vi "Set Clusters Visibility.vi"(4 "Normal Operation Control Cluster":refnum<vi>, 5 "Connection Status":T2, 6 "Connection Configuration Cluster":refnum<vi>, 8 "Error In":errorcluster, 9 "Control Type":T1, 10 "Normal Operation Indicator Cluster":refnum<vi>) -> (0 "Error Out":errorcluster, 1 "User Help":string, 3 "Control Type Out":T1)   [LabVIEW 2014]
doc: "Sets clusters visibility according to chosen mode for normal operation"
uses:
  Controls/Connection Status.ctl
  Controls/Controllers.ctl
  Controls/Controllers Clusters/Normal Operation Indicator Cluster.ctl
  Controls/User Help.ctl
  Controls/Controllers Clusters/Order in Normal Operation Control Cluster.ctl
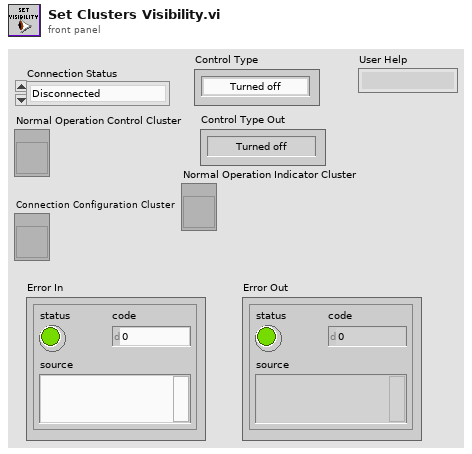
[diagram p1: front panel]
types:
  T1 = typedef "Controllers.ctl" = enum16{"Turned off", "Keyboard", "Mouse", "Pad", "Autonomous"}
  T2 = typedef "Connection Status.ctl" = enum16{"Disconnected", "Connected"}
  T3 = typedef "User Help.ctl" = enum16{"The Reaper Controller says hello!\nFirst you should establish connection with The Reaper.", "Connection established! Choose control mode.", "Something went wrong. Try another COM port.", "Disconnected. Do you want to connect again?", "Controls turned off", "Keyboard Mode", "Mouse Mode", "Pad Mode", "Autonomous Mode", "Unknown Operation occured", "Please connect before choosing control type!", "Settings available only if disconnected.", "Settings updated."}
  T4 = typedef "Order in Normal Operation Control Cluster.ctl" = enum16{"Disconnect Button", "Select Controller", "General Control Cluster ", "Game Pad Indicator Cluster", "Game Pad Control Cluster", "Mouse Control Cluster"}
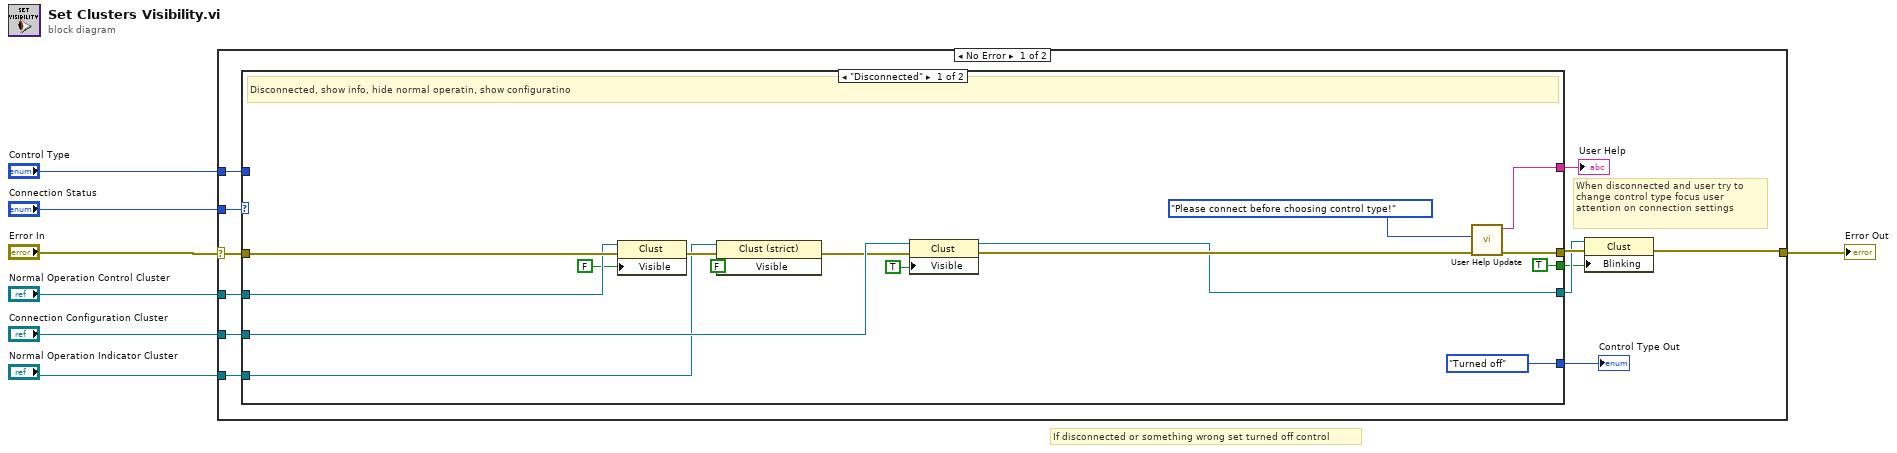
[diagram p0: block diagram]
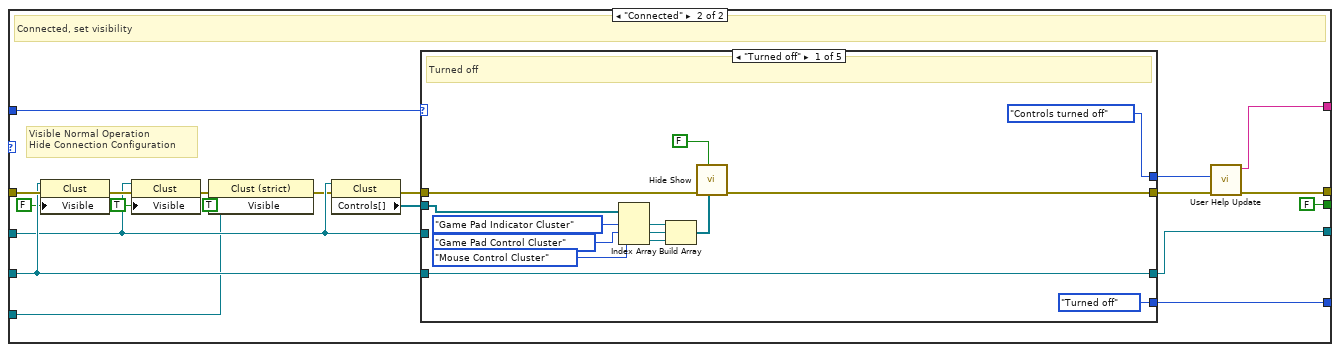
[diagram p2: hidden frame]
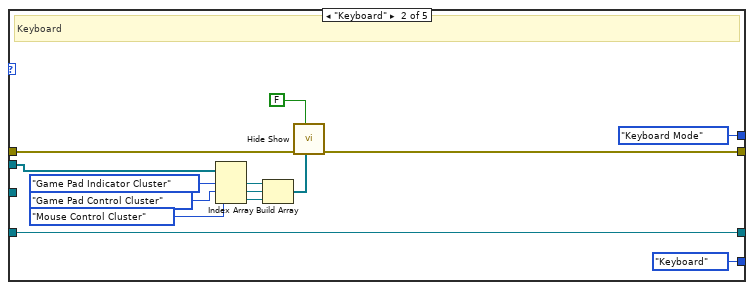
[diagram p3: hidden frame]
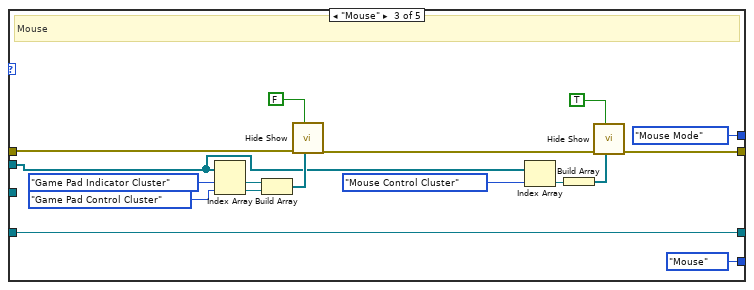
[diagram p4: hidden frame]
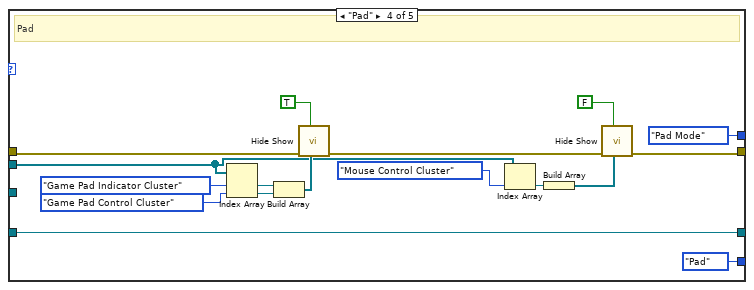
[diagram p5: hidden frame]
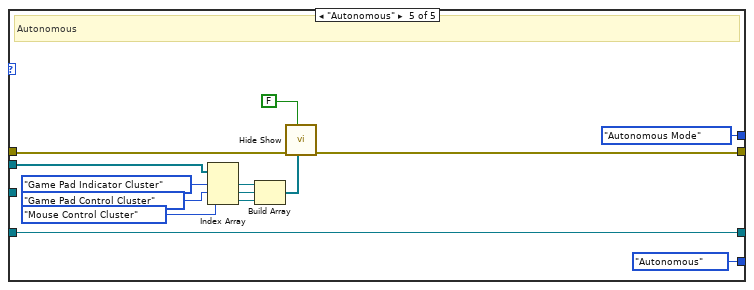
[diagram p6: hidden frame]
diagram:
  # "If disconnected or something wrong set turned off control"
  n1 = case shown="No Error" "Error In" {
    selector: "Error In" -> [w18 w132]
    tunnel: [w12 w132] -> w6
    tunnel: "Control Type" -> [w17 _]
    tunnel: "Connection Status" -> [w19 _]
    tunnel: "Normal Operation Control Cluster" -> [w16 _]
    tunnel: "Connection Configuration Cluster" -> [w15 _]
    tunnel: "Normal Operation Indicator Cluster" -> [w8 _]
    frame No Error {
      # "When disconnected and user try to change control type focus user attention on connection settings"
      n2 = case shown="\"Disconnected\"" w19 {
        tunnel: [w29 w53] -> w13
        tunnel: w18 -> [w35 w48]
        tunnel: w17 -> [_ w55]
        tunnel: w16 -> [w33 w42]
        tunnel: w15 -> [w34 w46]
        tunnel: [w30 w52] -> w14
        tunnel: [w26 w49] -> w11
        tunnel: [TRUE FALSE] -> w10
        tunnel: [Controllers."Turned off" ("Control Type") w43] -> w9
        tunnel: w8 -> [w20 w39]
        frame "Disconnected" {
          # "Disconnected, show info, hide normal operatin, show configuratino"
          n3 = property class="Clust"(reference=w33, error in=w35, "Visible"=FALSE) -> (error out=w23:errorcluster)  [unwired: 1 out]
          n4 = property class="Clust (strict)"(reference=w20, error in=w23, "Visible"=FALSE) -> (error out=w22:errorcluster)  [unwired: 1 out]
          n5 = property class="Clust"(reference=w34, error in=w22, "Visible"=TRUE) -> (reference out=w26:refnum<vi>, error out=w27:errorcluster)
          n6 = call "User Help Update.vi"("Error In"=w27, "Enum"=User_Help."Please connect before choosing control type!") -> ("Error Out"=w29:errorcluster, "User Help Out"=w30:string)  [unwired: 8 in]
        }
        frame "Connected" {
          # "Visible Normal Operation\nHide Connection Configuration"
          # "Connected, set visibility"
          n7 = property class="Clust"(reference=w46, error in=w48, "Visible"=FALSE) -> (error out=w47:errorcluster)  [unwired: 1 out]
          n8 = property class="Clust"(reference=w42, error in=w47, "Visible"=TRUE) -> (error out=w37:errorcluster)  [unwired: 1 out]
          n9 = property class="Clust (strict)"(reference=w39, error in=w37, "Visible"=TRUE) -> (error out=w36:errorcluster)  [unwired: 1 out]
          n10 = property class="Clust"(reference=w42, error in=w36) -> (error out=w41:errorcluster, "Controls[]"=w40:refnum<vi>[])  [unwired: 1 out]
          n11 = case shown="\"Turned off\"" w55 {
            tunnel: [w60 w75 w90 w106 w123] -> w54
            tunnel: w41 -> [w66 w76 w93 w110 w124]
            tunnel: w42 -> [_ _ _ _ _]
            tunnel: [User_Help."Controls turned off" ("Enum") User_Help."Keyboard Mode" ("Enum") User_Help."Mouse Mode" ("Enum") User_Help."Pad Mode" ("Enum") User_Help."Autonomous Mode" ("Enum")] -> w51
            tunnel: [w68 w82 w99 w116 w130] -> w49
            tunnel: w46 -> [w68 w82 w99 w116 w130]
            tunnel: [Controllers."Turned off" ("Control Type") Controllers."Keyboard" ("Control Type") Controllers."Mouse" ("Control Type") Controllers."Pad" ("Control Type") Controllers."Autonomous" ("Control Type")] -> w43
            tunnel: w40 -> [w65 w74 w85 w104 w122]
            frame "Turned off" {
              # "Turned off"
              n12 = Index Array(array=w65, index #1=Order_in_Normal_Operation_Control_Cluster."Game Pad Indicator Cluster" ("Order in Normal Operation Control Cluster"), index #2=Order_in_Normal_Operation_Control_Cluster."Game Pad Control Cluster" ("Order in Normal Operation Control Cluster"), index #3=Order_in_Normal_Operation_Control_Cluster."Mouse Control Cluster" ("Order in Normal Operation Control Cluster")) -> (element #1=w63:refnum<vi>, element #2=w58:refnum<vi>, element #3=w57:refnum<vi>)
              n13 = Build Array(w63, w58, w57) -> (w62:refnum<vi>[])
              n14 = call "Hide Show.vi"("Controls[]"=w62, "Visible?"=FALSE, "Error In"=w66) -> ("Error Out"=w60:errorcluster)  [unwired: 8 in]
            }
            frame "Keyboard" {
              # "Keyboard"
              n15 = Index Array(array=w74, index #1=Order_in_Normal_Operation_Control_Cluster."Game Pad Indicator Cluster" ("Order in Normal Operation Control Cluster"), index #2=Order_in_Normal_Operation_Control_Cluster."Game Pad Control Cluster" ("Order in Normal Operation Control Cluster"), index #3=Order_in_Normal_Operation_Control_Cluster."Mouse Control Cluster" ("Order in Normal Operation Control Cluster")) -> (element #1=w79:refnum<vi>, element #2=w72:refnum<vi>, element #3=w70:refnum<vi>)
              n16 = Build Array(w79, w72, w70) -> (w78:refnum<vi>[])
              n17 = call "Hide Show.vi"("Controls[]"=w78, "Visible?"=FALSE, "Error In"=w76) -> ("Error Out"=w75:errorcluster)  [unwired: 8 in]
            }
            frame "Mouse" {
              # "Mouse"
              n18 = Index Array(array=w85, index #1=Order_in_Normal_Operation_Control_Cluster."Game Pad Indicator Cluster" ("Order in Normal Operation Control Cluster"), index #2=Order_in_Normal_Operation_Control_Cluster."Game Pad Control Cluster" ("Order in Normal Operation Control Cluster")) -> (element #1=w96:refnum<vi>, element #2=w91:refnum<vi>)
              n19 = Build Array(w96, w91) -> (w95:refnum<vi>[])
              n20 = call "Hide Show.vi"("Controls[]"=w95, "Visible?"=FALSE, "Error In"=w93) -> ("Error Out"=w89:errorcluster)  [unwired: 8 in]
              n21 = Index Array(array=w85, index=Order_in_Normal_Operation_Control_Cluster."Mouse Control Cluster" ("Order in Normal Operation Control Cluster")) -> (element=w86:refnum<vi>)
              n22 = Build Array(w86) -> (w87:refnum<vi>[])
              n23 = call "Hide Show.vi"("Controls[]"=w87, "Visible?"=TRUE, "Error In"=w89) -> ("Error Out"=w90:errorcluster)  [unwired: 8 in]
            }
            frame "Pad" {
              # "Pad"
              n24 = Index Array(array=w104, index #1=Order_in_Normal_Operation_Control_Cluster."Game Pad Indicator Cluster" ("Order in Normal Operation Control Cluster"), index #2=Order_in_Normal_Operation_Control_Cluster."Game Pad Control Cluster" ("Order in Normal Operation Control Cluster")) -> (element #1=w113:refnum<vi>, element #2=w108:refnum<vi>)
              n25 = Build Array(w113, w108) -> (w112:refnum<vi>[])
              n26 = call "Hide Show.vi"("Controls[]"=w112, "Visible?"=TRUE, "Error In"=w110) -> ("Error Out"=w107:errorcluster)  [unwired: 8 in]
              n27 = Index Array(array=w104, index=Order_in_Normal_Operation_Control_Cluster."Mouse Control Cluster" ("Order in Normal Operation Control Cluster")) -> (element=w102:refnum<vi>)
              n28 = Build Array(w102) -> (w101:refnum<vi>[])
              n29 = call "Hide Show.vi"("Controls[]"=w101, "Visible?"=FALSE, "Error In"=w107) -> ("Error Out"=w106:errorcluster)  [unwired: 8 in]
            }
            frame "Autonomous" {
              # "Autonomous"
              n30 = Index Array(array=w122, index #1=Order_in_Normal_Operation_Control_Cluster."Game Pad Indicator Cluster" ("Order in Normal Operation Control Cluster"), index #2=Order_in_Normal_Operation_Control_Cluster."Game Pad Control Cluster" ("Order in Normal Operation Control Cluster"), index #3=Order_in_Normal_Operation_Control_Cluster."Mouse Control Cluster" ("Order in Normal Operation Control Cluster")) -> (element #1=w127:refnum<vi>, element #2=w120:refnum<vi>, element #3=w118:refnum<vi>)
              n31 = Build Array(w127, w120, w118) -> (w126:refnum<vi>[])
              n32 = call "Hide Show.vi"("Controls[]"=w126, "Visible?"=FALSE, "Error In"=w124) -> ("Error Out"=w123:errorcluster)  [unwired: 8 in]
            }
          }
          n33 = call "User Help Update.vi"("Error In"=w54, "Enum"=w51) -> ("Error Out"=w53:errorcluster, "User Help Out"=w52:string)  [unwired: 8 in]
        }
      }
      "User Help" <- w14
      "Control Type Out" <- w9
      n34 = property class="Clust"(reference=w11, error in=w13, "Blinking"=w10) -> (error out=w12:errorcluster)  [unwired: 1 out]
    }
    frame Error {
    }
  }
  "Error Out" <- w6
